vi "Close Device Core.vi"(8 "error in (no error)":errorcluster, 11 "CS++SimMotor in":refnum<class "CS++SimMotor.lvclass">) -> (0 "error out":errorcluster, 3 "CS++SimMotor out":refnum<class "CS++SimMotor.lvclass">)   [LabVIEW 2015, in "CS++SimMotor.lvlib" / "CS++SimMotor.lvclass"]
doc: "Close device driver connection."
uses:
  CS++SimMotor.lvclass
  CSPP_DeviceBase/CS++Motor/CS++Motor.lvclass
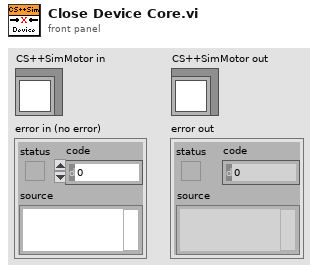
[diagram p1: front panel]
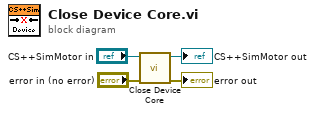
[diagram p0: block diagram]
diagram:
  n1 = call-parent "Close Device Core.vi"("error in (no error)"="error in (no error)", "CS++DeviceActor in"="CS++SimMotor in") -> ("error out"=→"error out":errorcluster, "CS++DeviceActor out"=→"CS++SimMotor out":refnum<class "CS++SimMotor.lvclass">)  [unwired: 8 in]
